vi "Deinitialize TCP Connection.vi"(11 "TCP Network Connection in":refnum<k5>) -> (0 "error out":errorcluster)   [LabVIEW 2023]
doc: "This VI is for deinitialization of TCP connection"
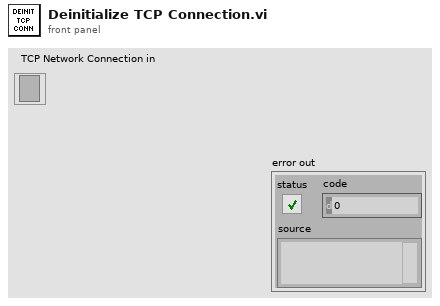
[diagram p1: front panel]
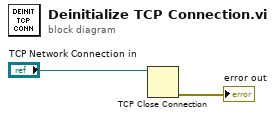
[diagram p0: block diagram]
diagram:
  n1 = TCP Close Connection(connection ID="TCP Network Connection in") -> (error out=→"error out":errorcluster)  [unwired: 2 in, 1 out]
